vi "Read Server RPC Methods.vi"(8 "error in (no error)":errorcluster, 11 "gRPC service in":refnum<class "ServiceName Template.lvclass">) -> (0 "error out":errorcluster, 2 "Server RPC Methods":T1, 3 "gRPC service out":refnum<class "ServiceName Template.lvclass">)   [LabVIEW 2019, in "ServiceName Template.lvclass"]
uses:
  ServiceName Template.lvclass
  gRPC lv Support/Shared/grpcId.ctl
  gRPC lv Support/grpc-lvsupport.lvlib
  gRPC lv Support/Server API/typeDefs/gRPCId Cluster.ctl
  typeDefs/Server gRPC UEs.ctl
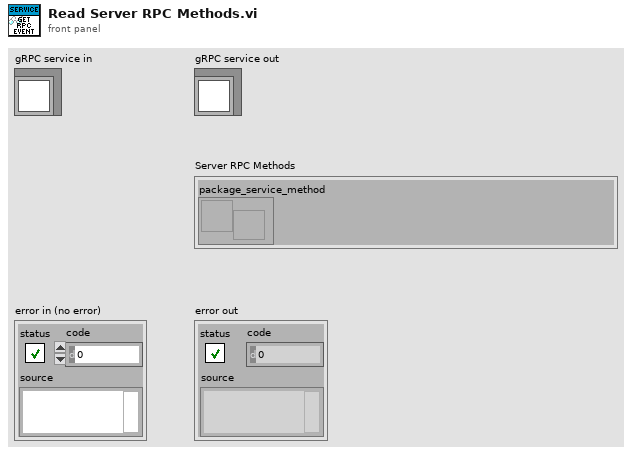
[diagram p1: front panel]
types:
  T1 = typedef "ServiceName Template.lvclass/Server gRPC UEs.ctl" = cluster{"package_service_method":refnum<user-event>}
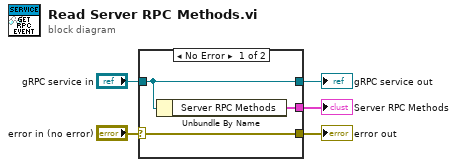
[diagram p0: block diagram]
diagram:
  n1 = case shown="No Error" "error in (no error)" {
    selector: "error in (no error)" -> [w8 w9]
    tunnel: [w8 w9] -> w4
    tunnel: [w7 w10] -> w2
    tunnel: "gRPC service in" -> [w7 w10]
    tunnel: [w6 _] -> w1
    frame No Error {
      n2 = Unbundle By Name(w7) -> ("Server RPC Methods"=w6:T1)
    }
    frame Error {
    }
  }
  "error out" <- w4
  "gRPC service out" <- w2
  "Server RPC Methods" <- w1
